vi "Periodic Tasks.vi"(8 "error in":errorcluster) -> ()   [LabVIEW 2019]
doc: "This VI runs in parallel to other tasks. It can contain as many user-defined periodic loops as you need. These can carry out PID or other sorts of timed response."
uses:
  <vilib>/Rock Robotics/WPI/ThirdParty/JAS_Junk/TrajLib/MatBuilder_Create.vi
  <vilib>/Rock Robotics/WPI/ThirdParty/JAS_Junk/TrajLib/Rotation_CreateAngle.vi
  <vilib>/Rock Robotics/WPI/ThirdParty/JAS_Junk/TrajLib/Conv_Deg_Radians.vi
  <vilib>/Rock Robotics/WPI/ThirdParty/JAS_Junk/TrajLib/LinearFilter_ResetToValue.vi
  <vilib>/Rock Robotics/WPI/ThirdParty/JAS_Junk/TrajLib/LinearFilter_Calculate.vi
  <vilib>/Rock Robotics/WPI/Utilities/WPI_GetSetVariantRefNum.vi
  Robot Global Data.vi
  <vilib>/Rock Robotics/WPI/ThirdParty/JAS_Junk/TrajLib/LinearFilter_MovingAverage.vi
  <vilib>/Rock Robotics/WPI/ThirdParty/JAS_Junk/TrajLib/LinearFilter_LowPassBW1.vi
  <vilib>/Rock Robotics/WPI/ThirdParty/JAS_Junk/TrajLib/LinearFilter_LowPassBW2.vi
  <vilib>/Rock Robotics/WPI/ThirdParty/JAS_Junk/TrajLib/LinearFilter_HighPassBW1.vi
  <vilib>/Rock Robotics/WPI/ThirdParty/JAS_Junk/TrajLib/LinearFilter_HighPassBW2.vi
  <vilib>/Rock Robotics/Network Tables/NT Write Number.vi
  <vilib>/Rock Robotics/WPI/ThirdParty/JAS_Junk/TrajLib/Trajectory_Library.lvlib
  <vilib>/NI_Real-Time Target Support.lvlib
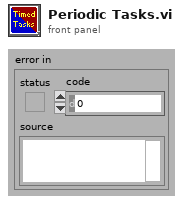
[diagram p1: front panel]
types:
  T1 = typedef "NI_Matrix.lvlib/RealMatrix.ctl" = dbl[][]
  T2 = typedef "Trajectory_Library.lvlib/POSE2D.ctl" = cluster{"TRANSLATION":T3, "ROTATION":T4}
  T3 = typedef "Trajectory_Library.lvlib/TRANSLATION2D.ctl" = cluster{"X":dbl, "Y":dbl}
  T4 = typedef "Trajectory_Library.lvlib/ROTATION2D.ctl" = cluster{"VALUE":dbl, "COS":dbl, "SIN":dbl}
  T5 = typedef "Trajectory_Library.lvlib/SWERVE_DRIVE_ODOMETRY.ctl" = cluster{"POSE":T2, "GyroOffset":T4, "PreviousAngle":T4, "PrevTime":dbl}
  T6 = typedef "Trajectory_Library.lvlib/SWERVE_DRIVE_KINEMATICS.ctl" = cluster{"NumModules":i32, "InverseKinematics":T1, "ForwardKinematics":T1, "Modules":T3[], "PrevCoR":T3}
  T7 = typedef "Trajectory_Library.lvlib/SWERVE_DRIVE_POSE_EST.ctl" = cluster{"M_VisionContR":T1, "m_nominal_dT":dbl, "m_PrevTime_Sec":dbl, "m_GyroOffset":T4, "m_PrevAngle":T4, "m_Observer":T8, "m_latencyCompensator":T11, "m_kinematics":T6}
  T8 = typedef "Trajectory_Library.lvlib/UNSCENTED_KALMAN_FILTER.ctl" = cluster{"m_P":T1, "m_xHat":T1, "States":i32, "Outputs":i32, "m_ContR":T1, "m_ContQ":T1, "m_SigmasF":T1, "m_dT_Sec":dbl, "MERWE_SCALED_SIGMA_PTS":T9, "meanFuncX":T10, "meanFuncY":T10, "residualFuncX":T10, "residualFuncY":T10, "addFuncX":T10, "addFuncXExtra":variant, "residualFuncYExtra":variant, "residualFuncXExtra":variant, "MeanFuncYExtra":variant, "MeanFuncXExtra":variant, "Inputs":i32}
  T9 = typedef "Trajectory_Library.lvlib/MERWE_SCALED_SIGMA_PTS.ctl" = cluster{"m_Wm":T1, "States":i32, "Alpha":dbl, "m_Wc":T1, "Kappa":i32}
  T10 = typedef "Trajectory_Library.lvlib/CALLBACK_FUNC_TYPE.ctl" = refnum<vi>
  T11 = typedef "Trajectory_Library.lvlib/KALMAN_FILTER_LATENCY_COMP.ctl" = cluster{"m_pastObserverSnapshots ":T12[]}
  T12 = typedef "Trajectory_Library.lvlib/OBSERVER_SNAP_LIST_ITEM.ctl" = cluster{"TimeStamp":dbl, "OBSERVER_SNAPSHOT":T13}
  T13 = typedef "Trajectory_Library.lvlib/OBSERVER_SNAPSHOT.ctl" = cluster{"ErrorCoVariance":T1, "xHat":T1, "LocalMeasurements":T1, "Inputs":T1}
  T14 = enum16{"Moving Average", "Low Pass 1st Order Butterworth", "Low Pass 2nd Order Butterworth", "High Pass 1st Order Butterworth", "High Pass 2nd Order Butterworth"}
  T15 = typedef "Trajectory_Library.lvlib/SWERVE_DRIVE_MODULE_STATE.ctl" = cluster{"Speed":dbl, "Angle":T4}
  T16 = typedef "NI_Real-Time Target Support.lvlib/RT CPU Load.ctl" = cluster{"Total (%)":dbl, "Time Critical (%)":dbl, "Timed Structures (%)":dbl, "High (%)":dbl, "Above Normal (%)":dbl, "Normal (%)":dbl, "Background (%)":dbl, "Idle (%)":dbl, "ISR (%)":dbl}
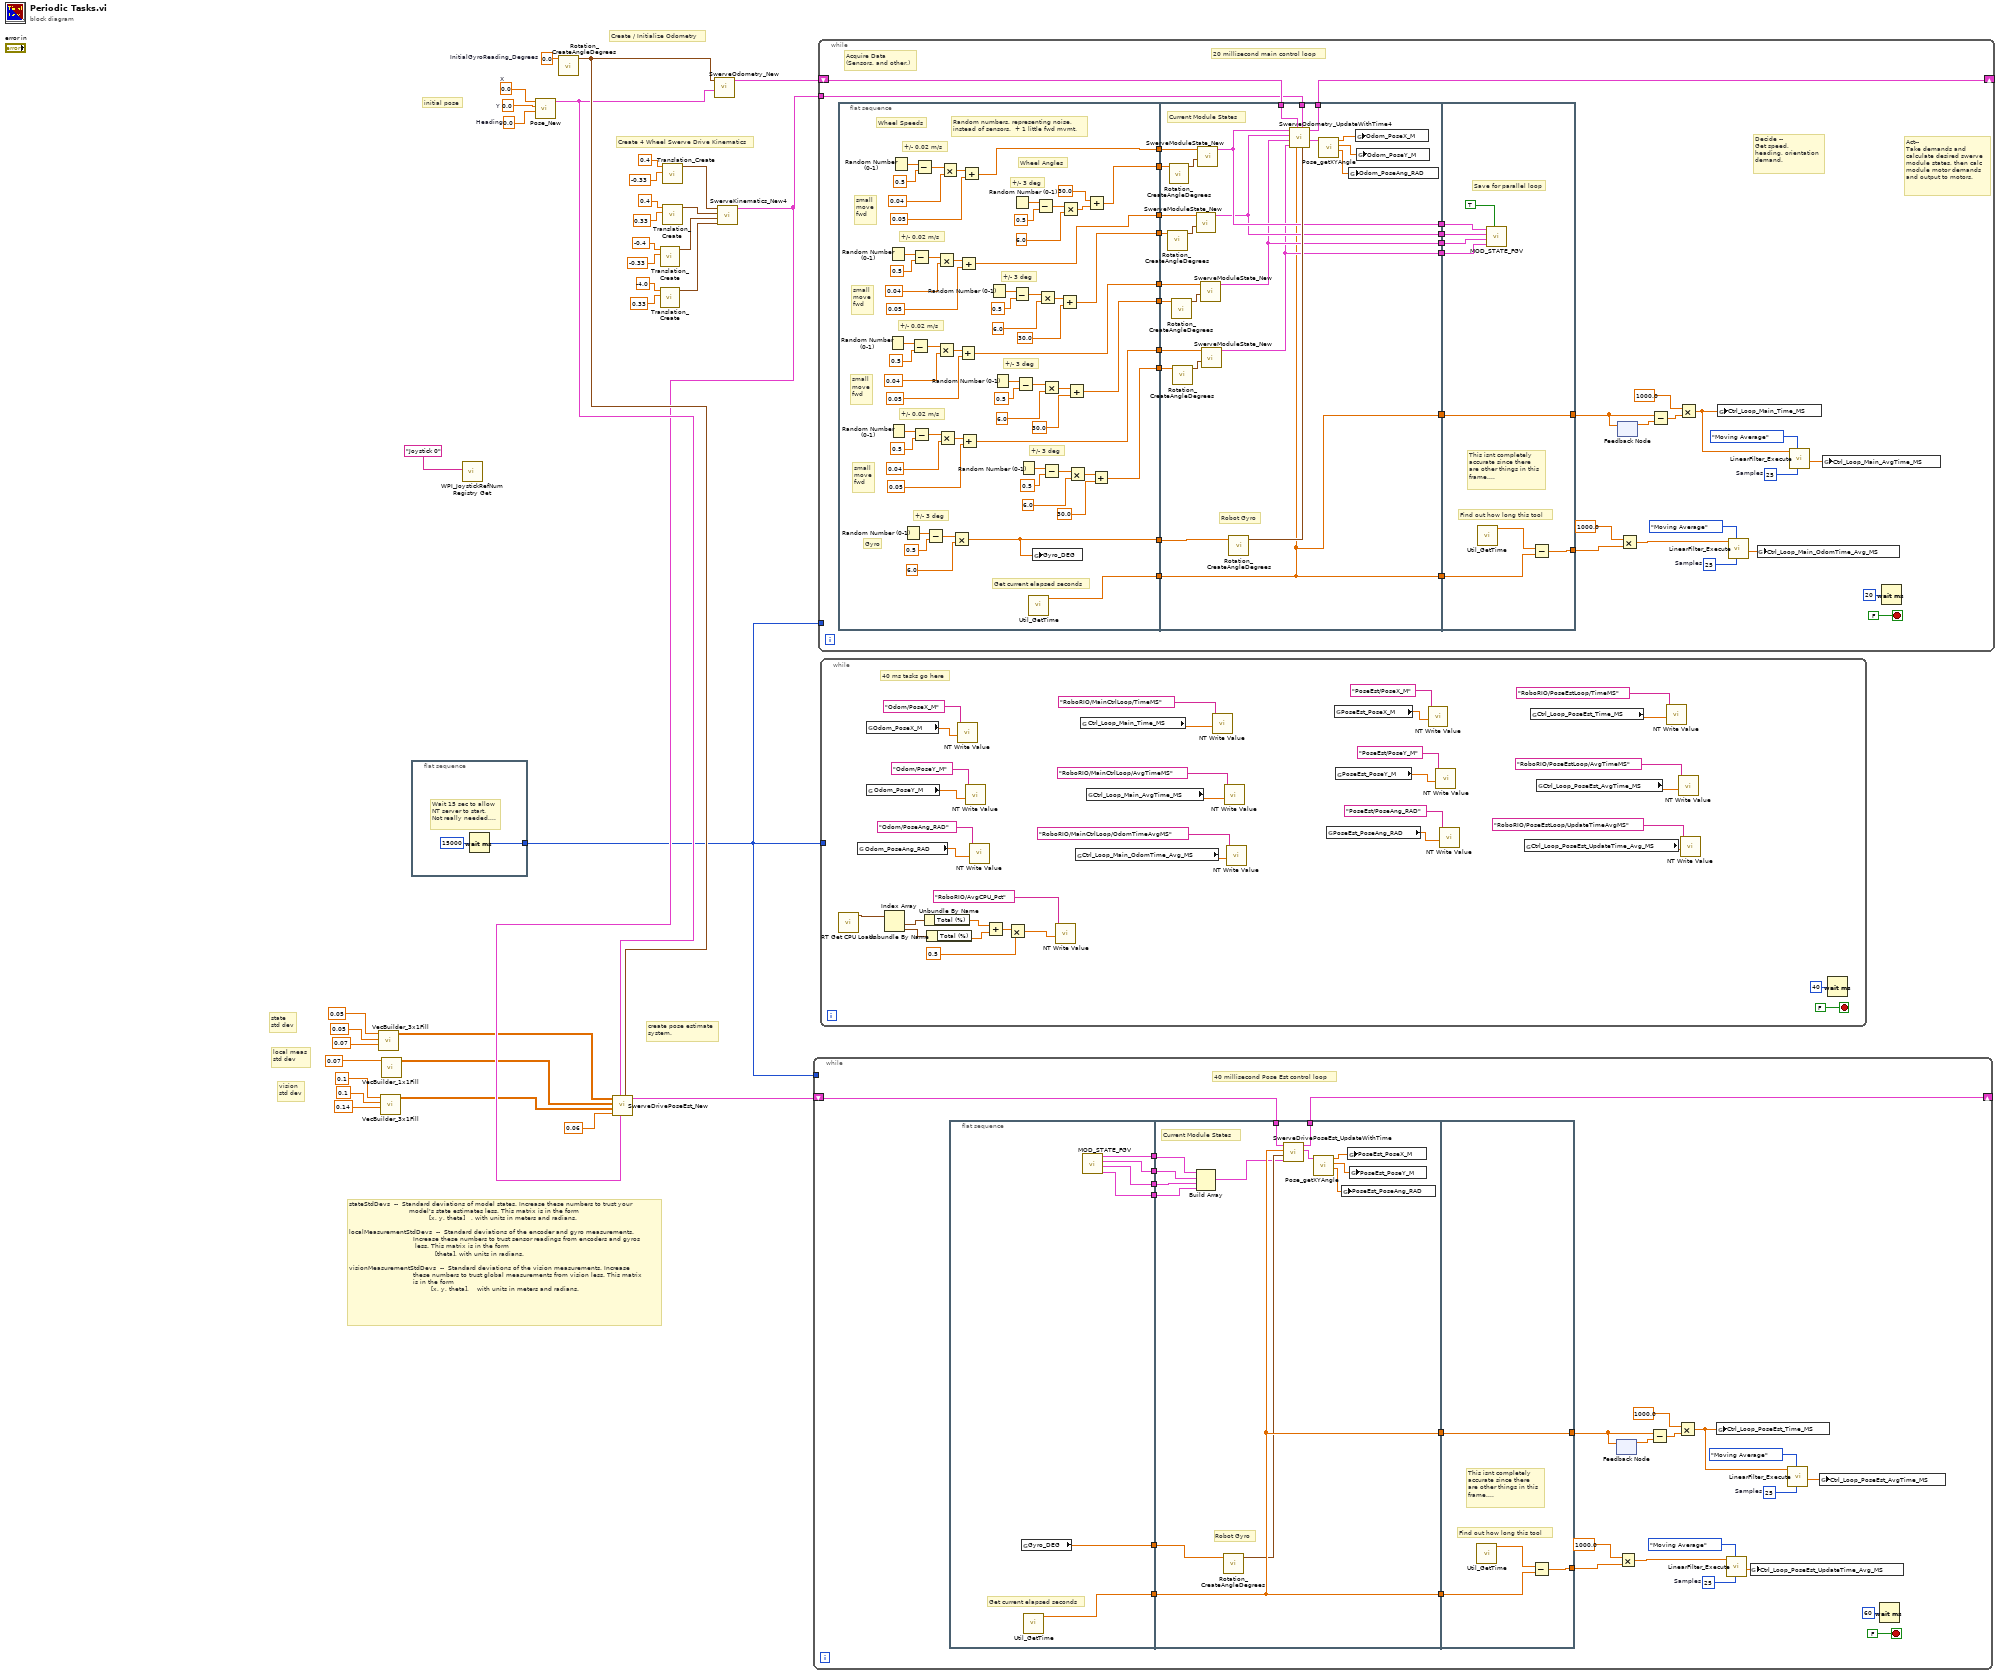
[diagram p0: block diagram]
diagram:
  w18 = 0.0  # X
  w19 = 0.0  # Y
  w20 = 0.0  # Heading
  w21 = 0.0  # InitialGyroReading_Degrees
  # "stateStdDevs  --  Standard deviations of model states. Increase these numbers to trust your\n                              model's state estimates less. This matrix is in the form \n                                        [x, y, theta]   , with units in meters and radians.\n\nlocalMeasurementStdDevs  --  Standard deviations of the encoder and gyro measurements.\n                                Increase these numbers to trust sensor readings from encoders and gyros \n                                 less. This matrix is in the form \n                                           [theta], with units in radians.\n\nvisionMeasurementStdDevs  --  Standard deviations of the vision measurements. Increase \n                                these numbers to trust global measurements from vision less. This matrix \n                                is in the form \n                                         [x, y, theta],    with units in meters and radians."
  # "vision \nstd dev"
  # "local meas\nstd dev"
  # "state\nstd dev"
  # "create pose estimate\nsystem."
  # "initial pose"
  # "Create / Initialize Odometry"
  # "Create 4 Wheel Swerve Drive Kinematics"
  n1 = call <vilib>:"VecBuilder_3x1Fill.vi"("R2"=0.07 ("element"), "R1"=0.05 ("element"), "R0"=0.05 ("element")) -> ("output matrix"=w4:T1)  [unwired: 8 in]
  n2 = call <vilib>:"VecBuilder_3x1Fill.vi"("R2"=0.14 ("element"), "R1"=0.1 ("element"), "R0"=0.1 ("element")) -> ("output matrix"=w2:T1)  [unwired: 8 in]
  n3 = call <vilib>:"VecBuilder_1x1Fill.vi"("R0_C0"=0.07 ("element")) -> ("output matrix"=w3:T1)  [unwired: 10 in]
  n4 = flat-sequence {
    tunnel: [w35] -> w1
    frame #0 {
      # "Wait 15 sec to allow\nNT server to start.\nNot really needed...."
      n5 = Wait (ms)(milliseconds to wait=u32 15000) -> (millisecond timer value=w35:u32)
    }
  }
  n6 = call <vilib>:"WPI_JoystickRefNum Registry Get.vi"("refnum name"="Joystick 0") -> ()  [unwired: 1 in, 10 out]
  n7 = call <vilib>:"Pose_New.vi"("Heading"=w20, "Y"=w19, "X"=w18) -> ("out POSe"=w15:T2)  [unwired: 8 in]
  n8 = call <vilib>:"Rotation_CreateAngleDegrees.vi"("Angle_Degrees"=w21) -> ("ROTATION"=w16:T4)  [unwired: 10 in]
  n9 = call <vilib>:"Translation_Create.vi"("Y"=-0.33, "X"=-0.4) -> ("TRANSLATION"=w23:T3)  [unwired: 9 in]
  n10 = call <vilib>:"Translation_Create.vi"("Y"=0.33, "X"=-4.0) -> ("TRANSLATION"=w22:T3)  [unwired: 9 in]
  n11 = call <vilib>:"Translation_Create.vi"("Y"=-0.33, "X"=0.4) -> ("TRANSLATION"=w25:T3)  [unwired: 9 in]
  n12 = call <vilib>:"Translation_Create.vi"("Y"=0.33, "X"=0.4) -> ("TRANSLATION"=w24:T3)  [unwired: 9 in]
  n13 = call <vilib>:"SwerveOdometry_New.vi"("InitialPose"=w15, "gyroAngle"=w16) -> ("SWERVE_DRIVE_ODOMETRY"=w17:T5)  [unwired: 9 in]
  n14 = call <vilib>:"SwerveKinematics_New4.vi"("wheel 3"=w22, "wheel 2"=w23, "wheel 1"=w24, "wheel 0"=w25) -> ("SWERVE_DRIVE_KINEMATICS"=w13:T6)  [unwired: 7 in]
  n15 = call <vilib>:"SwerveDrivePoseEst_New.vi"("gyroAngle"=w16, "SwerveKinematics"=w13, "InitialPose"=w15, "dt_Seconds"=0.06, "VisionMeasurementStdDevs"=w2, "LocalMeasurementStdDevs"=w3, "StateStdDevs"=w4) -> ("SwerveDrivePoseEstimate"=w12:T7)  [unwired: 3 in, 1 out]
  n16 = while {
    shift-right: [w37] -> _
    shift-left: w12 -> [w60]
    tunnel: w1 -> [_]
    stop <- FALSE stop-if-true
    w46 = 25  # Samples
    w56 = 25  # Samples
    # "40 millisecond Pose Est control loop"
    n17 = flat-sequence {
      tunnel: [w68] -> w51
      tunnel: [w67] -> w42
      tunnel: [w66] -> w41
      tunnel: [w65] -> w40
      tunnel: [w64] -> w39
      tunnel: [w63] -> w38
      tunnel: w60 -> [w74]
      tunnel: w51 -> [w73]
      tunnel: [w73] -> w50
      tunnel: [w73] -> w49
      tunnel: w42 -> [w78]
      tunnel: w41 -> [w77]
      tunnel: w40 -> [w76]
      tunnel: w39 -> [w75]
      tunnel: w38 -> [w79]
      tunnel: [w69] -> w37
      tunnel: [w86] -> w52
      tunnel: w50 -> [w86]
      tunnel: w49 -> [w84]
      tunnel: [w83] -> w47
      frame #0 {
        # "Get current elapsed seconds"
        n18 = global read "Robot Global Data.vi" "Gyro_DEG"() -> (w63:dbl)
        n19 = call <vilib>:"Util_GetTime.vi"() -> ("FPGA_Time_Seconds"=w68:dbl)  [unwired: 10 in, 1 out]
        n20 = call "MOD_STATE_FGV.vi"() -> ("outMS3"=w64:T15, "outMS2"=w65:T15, "outMS1"=w66:T15, "outMS0"=w67:T15)  [unwired: 8 in]
      }
      frame #1 {
        # "Current Module States"
        # "Robot Gyro"
        n21 = Build Array(w78, w77, w76, w75) -> (w71:T15[])
        n22 = call <vilib>:"Rotation_CreateAngleDegrees.vi"("Angle_Degrees"=w79) -> ("ROTATION"=w72:T4)  [unwired: 10 in]
        n23 = call <vilib>:"SwerveDrivePoseEst_UpdateWithTime.vi"("SweveModuleStates"=w71, "GyroAngle"=w72, "CurrentTimeSeconds"=w73, "in SwerveDrivePoseEstimate"=w74) -> ("Estimated Pose"=w70:T2, "Out SwerveDrivePoseEstimate"=w69:T7)  [unwired: 5 in, 1 out]
        n24 = call <vilib>:"Pose_getXYAngle.vi"("in POSE"=w70) -> ("Angle"=w80:dbl, "Y"=w81:dbl, "X"=w82:dbl)  [unwired: 8 in]
        n25 = global write "Robot Global Data.vi" "PoseEst_PoseAng_RAD"(w80) -> ()
        n26 = global write "Robot Global Data.vi" "PoseEst_PoseX_M"(w82) -> ()
        n27 = global write "Robot Global Data.vi" "PoseEst_PoseY_M"(w81) -> ()
      }
      frame #2 {
        # "This isnt completely\naccurate since there\nare other things in this\nframe...."
        # "Find out how long this tool"
        n28 = call <vilib>:"Util_GetTime.vi"() -> ("FPGA_Time_Seconds"=w85:dbl)  [unwired: 10 in, 1 out]
        n29 = Subtract(x=w85, y=w84) -> (x-y=w83:dbl)
      }
    }
    n30 = feedback-in #1(w52) -> ()
    n31 = feedback #1() -> (w59:dbl)  [unwired: 1 in]
    n32 = Multiply(x=1000.0, y=w47) -> (x*y=w44:dbl)
    n33 = Subtract(x=w52, y=w59) -> (x-y=w58:dbl)
    n34 = Multiply(x=1000.0, y=w58) -> (x*y=w54:dbl)
    n35 = global write "Robot Global Data.vi" "Ctrl_Loop_PoseEst_Time_MS"(w54) -> ()
    n36 = call <vilib>:"LinearFilter_Execute.vi"("Samples"=w46, "Filter Type"=T14."Moving Average", "Input"=w44) -> ("Output"=w43:dbl)  [unwired: 7 in, 1 out]
    n37 = global write "Robot Global Data.vi" "Ctrl_Loop_PoseEst_UpdateTime_Avg_MS"(w43) -> ()
    n38 = call <vilib>:"LinearFilter_Execute.vi"("Samples"=w56, "Filter Type"=T14."Moving Average", "Input"=w54) -> ("Output"=w53:dbl)  [unwired: 7 in, 1 out]
    n39 = global write "Robot Global Data.vi" "Ctrl_Loop_PoseEst_AvgTime_MS"(w53) -> ()
    n40 = Wait (ms)(milliseconds to wait=u32 60) -> ()  [unwired: 1 out]
  }
  n41 = while {
    shift-right: [w117] -> _
    shift-left: w17 -> [w119]
    tunnel: w13 -> [w118]
    tunnel: w1 -> [_]
    stop <- FALSE stop-if-true
    w90 = 25  # Samples
    w113 = 25  # Samples
    # "Act--\nTake demands and \ncalculate desired swerve\nmodule states, then calc\nmodule motor demands\nand output to motors."
    # "Decide -- \nGet speed,\nheading, orientation\ndemand."
    # "Acquire Data\n(Sensors, and other.)"
    # "20 millisecond main control loop"
    n42 = flat-sequence {
      tunnel: [w132] -> w108
      tunnel: [w129] -> w107
      tunnel: [w125] -> w106
      tunnel: [w124] -> w105
      tunnel: [w134] -> w104
      tunnel: [w183] -> w103
      tunnel: [w138] -> w102
      tunnel: [w137] -> w101
      tunnel: [w136] -> w100
      tunnel: [w135] -> w99
      tunnel: w119 -> [w205]
      tunnel: w118 -> [w204]
      tunnel: [w197] -> w117
      tunnel: w108 -> [w203]
      tunnel: w107 -> [w202]
      tunnel: w106 -> [w201]
      tunnel: w105 -> [w200]
      tunnel: w104 -> [w199]
      tunnel: w103 -> [w184]
      tunnel: w102 -> [w188]
      tunnel: w101 -> [w187]
      tunnel: w100 -> [w186]
      tunnel: w99 -> [w185]
      tunnel: [w192] -> w98
      tunnel: [w191] -> w97
      tunnel: [w190] -> w96
      tunnel: [w189] -> w95
      tunnel: [w184] -> w94
      tunnel: [w184] -> w93
      tunnel: [w218] -> w109
      tunnel: w98 -> [w213]
      tunnel: w97 -> [w214]
      tunnel: w96 -> [w215]
      tunnel: w95 -> [w216]
      tunnel: w94 -> [w218]
      tunnel: w93 -> [w211]
      tunnel: [w210] -> w91
      frame #0 {
        # "small\nmove\nfwd"
        # "+/- 0.02 m/s"
        # "small\nmove\nfwd"
        # "+/- 0.02 m/s"
        # "small\nmove\nfwd"
        # "+/- 0.02 m/s"
        # "small\nmove\nfwd"
        # "+/- 0.02 m/s"
        # "Wheel Speeds"
        # "Random numbers, representing noise,\ninstead of sensors.  + 1 little fwd mvmt."
        # "Gyro"
        # "+/- 3 deg"
        # "+/- 3 deg"
        # "+/- 3 deg"
        # "+/- 3 deg"
        # "+/- 3 deg"
        # "Wheel Angles"
        # "Get current elapsed seconds"
        n43 = Random Number (0-1)() -> (number: 0 to 1=w157:dbl)
        n44 = Random Number (0-1)() -> (number: 0 to 1=w154:dbl)
        n45 = Random Number (0-1)() -> (number: 0 to 1=w160:dbl)
        n46 = Random Number (0-1)() -> (number: 0 to 1=w151:dbl)
        n47 = Random Number (0-1)() -> (number: 0 to 1=w165:dbl)
        n48 = Subtract(x=w157, y=0.5) -> (x-y=w158:dbl)
        n49 = Subtract(x=w154, y=0.5) -> (x-y=w155:dbl)
        n50 = Subtract(x=w160, y=0.5) -> (x-y=w161:dbl)
        n51 = Subtract(x=w151, y=0.5) -> (x-y=w152:dbl)
        n52 = Subtract(x=w165, y=0.5) -> (x-y=w166:dbl)
        n53 = Multiply(x=w158, y=0.04) -> (x*y=w159:dbl)
        n54 = Multiply(x=w155, y=0.04) -> (x*y=w156:dbl)
        n55 = Multiply(x=w161, y=0.04) -> (x*y=w162:dbl)
        n56 = Multiply(x=w152, y=0.04) -> (x*y=w153:dbl)
        n57 = Multiply(x=w166, y=6.0) -> (x*y=w134:dbl)
        n58 = Add(x=w159, y=0.05) -> (x+y=w136:dbl)
        n59 = Add(x=w156, y=0.05) -> (x+y=w137:dbl)
        n60 = Add(x=w162, y=0.05) -> (x+y=w135:dbl)
        n61 = Add(x=w153, y=0.05) -> (x+y=w138:dbl)
        n62 = Random Number (0-1)() -> (number: 0 to 1=w177:dbl)
        n63 = Random Number (0-1)() -> (number: 0 to 1=w179:dbl)
        n64 = Random Number (0-1)() -> (number: 0 to 1=w175:dbl)
        n65 = Subtract(x=w177, y=0.5) -> (x-y=w178:dbl)
        n66 = Subtract(x=w179, y=0.5) -> (x-y=w180:dbl)
        n67 = Random Number (0-1)() -> (number: 0 to 1=w181:dbl)
        n68 = call <vilib>:"Util_GetTime.vi"() -> ("FPGA_Time_Seconds"=w183:dbl)  [unwired: 10 in, 1 out]
        n69 = global write "Robot Global Data.vi" "Gyro_DEG"(w134) -> ()
        n70 = Subtract(x=w175, y=0.5) -> (x-y=w176:dbl)
        n71 = Multiply(x=w178, y=6.0) -> (x*y=w130:dbl)
        n72 = Multiply(x=w180, y=6.0) -> (x*y=w127:dbl)
        n73 = Subtract(x=w181, y=0.5) -> (x-y=w182:dbl)
        n74 = Add(x=w130, y=30.0) -> (x+y=w129:dbl)
        n75 = Multiply(x=w176, y=6.0) -> (x*y=w133:dbl)
        n76 = Add(x=w127, y=30.0) -> (x+y=w125:dbl)
        n77 = Multiply(x=w182, y=6.0) -> (x*y=w123:dbl)
        n78 = Add(x=30.0, y=w133) -> (x+y=w132:dbl)
        n79 = Add(x=w123, y=30.0) -> (x+y=w124:dbl)
      }
      frame #1 {
        # "Current Module States"
        # "Robot Gyro"
        n80 = call <vilib>:"Rotation_CreateAngleDegrees.vi"("Angle_Degrees"=w202) -> ("ROTATION"=w208:T4)  [unwired: 10 in]
        n81 = call <vilib>:"Rotation_CreateAngleDegrees.vi"("Angle_Degrees"=w203) -> ("ROTATION"=w209:T4)  [unwired: 10 in]
        n82 = call <vilib>:"Rotation_CreateAngleDegrees.vi"("Angle_Degrees"=w201) -> ("ROTATION"=w207:T4)  [unwired: 10 in]
        n83 = call <vilib>:"Rotation_CreateAngleDegrees.vi"("Angle_Degrees"=w200) -> ("ROTATION"=w206:T4)  [unwired: 10 in]
        n84 = call <vilib>:"SwerveModuleState_New.vi"("ROTATION"=w208, "Speed"=w187) -> ("SWERVE_DRIVE_MODULE_STATE"=w191:T15)  [unwired: 9 in]
        n85 = call <vilib>:"SwerveModuleState_New.vi"("ROTATION"=w209, "Speed"=w188) -> ("SWERVE_DRIVE_MODULE_STATE"=w192:T15)  [unwired: 9 in]
        n86 = call <vilib>:"SwerveModuleState_New.vi"("ROTATION"=w207, "Speed"=w186) -> ("SWERVE_DRIVE_MODULE_STATE"=w190:T15)  [unwired: 9 in]
        n87 = call <vilib>:"SwerveModuleState_New.vi"("ROTATION"=w206, "Speed"=w185) -> ("SWERVE_DRIVE_MODULE_STATE"=w189:T15)  [unwired: 9 in]
        n88 = call <vilib>:"Rotation_CreateAngleDegrees.vi"("Angle_Degrees"=w199) -> ("ROTATION"=w198:T4)  [unwired: 10 in]
        n89 = call <vilib>:"SwerveOdometry_UpdateWithTime4.vi"("gyroAngle"=w198, "SWERVE_DRIVE_KINEMATICS"=w204, "Time"=w184, "in SWERVE_DRIVE_ODOMETRY"=w205, "Wheel State 3"=w189, "Wheel State 2"=w190, "Wheel State 1"=w191, "Wheel State 0"=w192) -> ("robot POSE"=w196:T2, "out SWERVE_DRIVE_ODOMETRY"=w197:T5)  [unwired: 2 in]
        n90 = call <vilib>:"Pose_getXYAngle.vi"("in POSE"=w196) -> ("Angle"=w193:dbl, "Y"=w194:dbl, "X"=w195:dbl)  [unwired: 8 in]
        n91 = global write "Robot Global Data.vi" "Odom_PoseAng_RAD"(w193) -> ()
        n92 = global write "Robot Global Data.vi" "Odom_PoseX_M"(w195) -> ()
        n93 = global write "Robot Global Data.vi" "Odom_PoseY_M"(w194) -> ()
      }
      frame #2 {
        # "This isnt completely\naccurate since there\nare other things in this\nframe...."
        # "Find out how long this tool"
        # "Save for parallel loop"
        n94 = call <vilib>:"Util_GetTime.vi"() -> ("FPGA_Time_Seconds"=w212:dbl)  [unwired: 10 in, 1 out]
        n95 = call "MOD_STATE_FGV.vi"("Write"=TRUE, "inMS3"=w216, "inMS2"=w215, "inMS1"=w214, "inMS0"=w213) -> ()  [unwired: 3 in, 4 out]
        n96 = Subtract(x=w212, y=w211) -> (x-y=w210:dbl)
      }
    }
    n97 = feedback-in #2(w109) -> ()
    n98 = feedback #2() -> (w116:dbl)  [unwired: 1 in]
    n99 = Multiply(x=1000.0, y=w91) -> (x*y=w88:dbl)
    n100 = Subtract(x=w109, y=w116) -> (x-y=w115:dbl)
    n101 = Multiply(x=1000.0, y=w115) -> (x*y=w111:dbl)
    n102 = global write "Robot Global Data.vi" "Ctrl_Loop_Main_Time_MS"(w111) -> ()
    n103 = call <vilib>:"LinearFilter_Execute.vi"("Samples"=w90, "Filter Type"=T14."Moving Average", "Input"=w88) -> ("Output"=w87:dbl)  [unwired: 7 in, 1 out]
    n104 = global write "Robot Global Data.vi" "Ctrl_Loop_Main_OdomTime_Avg_MS"(w87) -> ()
    n105 = call <vilib>:"LinearFilter_Execute.vi"("Samples"=w113, "Filter Type"=T14."Moving Average", "Input"=w111) -> ("Output"=w110:dbl)  [unwired: 7 in, 1 out]
    n106 = global write "Robot Global Data.vi" "Ctrl_Loop_Main_AvgTime_MS"(w110) -> ()
    n107 = Wait (ms)(milliseconds to wait=u32 20) -> ()  [unwired: 1 out]
  }
  n108 = while {
    tunnel: w1 -> [_]
    stop <- FALSE stop-if-true
    # "40 ms tasks go here"
    n109 = call <vilib>:"RT Get CPU Loads.vi"() -> ("CPU loads"=w245:T16[])  [unwired: 10 in, 1 out]
    n110 = global read "Robot Global Data.vi" "Odom_PoseAng_RAD"() -> (w246:dbl)
    n111 = global read "Robot Global Data.vi" "Odom_PoseX_M"() -> (w250:dbl)
    n112 = global read "Robot Global Data.vi" "Odom_PoseY_M"() -> (w247:dbl)
    n113 = Index Array(array=w245) -> (element #1=w244:T16, element #2=w243:T16)  [unwired: 2 in]
    n114 = Unbundle By Name(w244) -> ("Total (%)"=w242:dbl)
    n115 = Unbundle By Name(w243) -> ("Total (%)"=w241:dbl)
    n116 = call-poly <vilib>:"NT Write Value.vi"("Numeric"=w250, "Name"="Odom/PoseX_M") -> ()  [unwired: 9 in, 1 out]
    n117 = call-poly <vilib>:"NT Write Value.vi"("Numeric"=w247, "Name"="Odom/PoseY_M") -> ()  [unwired: 9 in, 1 out]
    n118 = call-poly <vilib>:"NT Write Value.vi"("Numeric"=w246, "Name"="Odom/PoseAng_RAD") -> ()  [unwired: 9 in, 1 out]
    n119 = Add(x=w242, y=w241) -> (x+y=w240:dbl)
    n120 = Multiply(x=w240, y=0.5) -> (x*y=w237:dbl)
    n121 = call-poly <vilib>:"NT Write Value.vi"("Numeric"=w237, "Name"="RoboRIO/AvgCPU_Pct") -> ()  [unwired: 9 in, 1 out]
    n122 = global read "Robot Global Data.vi" "Ctrl_Loop_Main_OdomTime_Avg_MS"() -> (w231:dbl)
    n123 = global read "Robot Global Data.vi" "Ctrl_Loop_Main_Time_MS"() -> (w235:dbl)
    n124 = global read "Robot Global Data.vi" "Ctrl_Loop_Main_AvgTime_MS"() -> (w233:dbl)
    n125 = call-poly <vilib>:"NT Write Value.vi"("Numeric"=w235, "Name"="RoboRIO/MainCtrlLoop/TimeMS") -> ()  [unwired: 9 in, 1 out]
    n126 = call-poly <vilib>:"NT Write Value.vi"("Numeric"=w233, "Name"="RoboRIO/MainCtrlLoop/AvgTimeMS") -> ()  [unwired: 9 in, 1 out]
    n127 = call-poly <vilib>:"NT Write Value.vi"("Numeric"=w231, "Name"="RoboRIO/MainCtrlLoop/OdomTimeAvgMS") -> ()  [unwired: 9 in, 1 out]
    n128 = global read "Robot Global Data.vi" "PoseEst_PoseAng_RAD"() -> (w225:dbl)
    n129 = global read "Robot Global Data.vi" "PoseEst_PoseX_M"() -> (w229:dbl)
    n130 = global read "Robot Global Data.vi" "PoseEst_PoseY_M"() -> (w226:dbl)
    n131 = call-poly <vilib>:"NT Write Value.vi"("Numeric"=w229, "Name"="PoseEst/PoseX_M") -> ()  [unwired: 9 in, 1 out]
    n132 = call-poly <vilib>:"NT Write Value.vi"("Numeric"=w226, "Name"="PoseEst/PoseY_M") -> ()  [unwired: 9 in, 1 out]
    n133 = call-poly <vilib>:"NT Write Value.vi"("Numeric"=w225, "Name"="PoseEst/PoseAng_RAD") -> ()  [unwired: 9 in, 1 out]
    n134 = global read "Robot Global Data.vi" "Ctrl_Loop_PoseEst_UpdateTime_Avg_MS"() -> (w219:dbl)
    n135 = global read "Robot Global Data.vi" "Ctrl_Loop_PoseEst_Time_MS"() -> (w223:dbl)
    n136 = global read "Robot Global Data.vi" "Ctrl_Loop_PoseEst_AvgTime_MS"() -> (w221:dbl)
    n137 = call-poly <vilib>:"NT Write Value.vi"("Numeric"=w223, "Name"="RoboRIO/PoseEstLoop/TimeMS") -> ()  [unwired: 9 in, 1 out]
    n138 = call-poly <vilib>:"NT Write Value.vi"("Numeric"=w221, "Name"="RoboRIO/PoseEstLoop/AvgTimeMS") -> ()  [unwired: 9 in, 1 out]
    n139 = call-poly <vilib>:"NT Write Value.vi"("Numeric"=w219, "Name"="RoboRIO/PoseEstLoop/UpdateTimeAvgMS") -> ()  [unwired: 9 in, 1 out]
    n140 = Wait (ms)(milliseconds to wait=u32 40) -> ()  [unwired: 1 out]
  }
